vi "AutoFeed_Back.vi"(9 "error":errorcluster, 10 "Time (ms)":i32, 11 "State":dbl) -> (3 "Feedback_State":cluster{"Time_Met":bool, "error ":errorcluster})   [LabVIEW 2015]
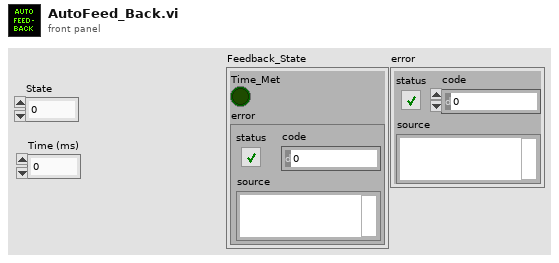
[diagram p1: front panel]
types:
  T1 = enum16{"Standard", "Momentary Falling", "Momentary Rising", "Momentary Falling and Rising"}
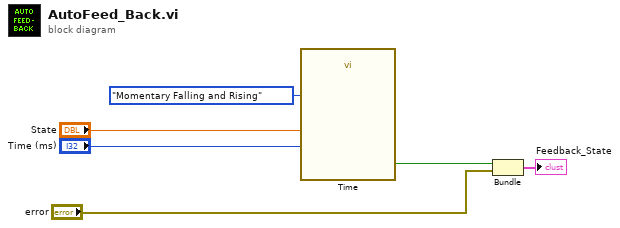
[diagram p0: block diagram]
diagram:
  n1 = call "Time.vi"("Reset_Int"="State", "Configuration"=T1."Momentary Falling and Rising", "Time_Limit  (ms)"="Time (ms)") -> ("Time_Met"=w6:bool)  [unwired: 8 in]
  n2 = Bundle("Time_Met"=w6, "error"="error") -> (→"Feedback_State":cluster{"Time_Met":bool, "error ":errorcluster})  [unwired: 1 in]
